vi "Read Com.vi"() -> ()   [LabVIEW 2016]
panel:
  in  "Boolean":bool
  out "Waveform Chart":dbl(graph)
  in  "stop":bool
  out "concatenated string":string
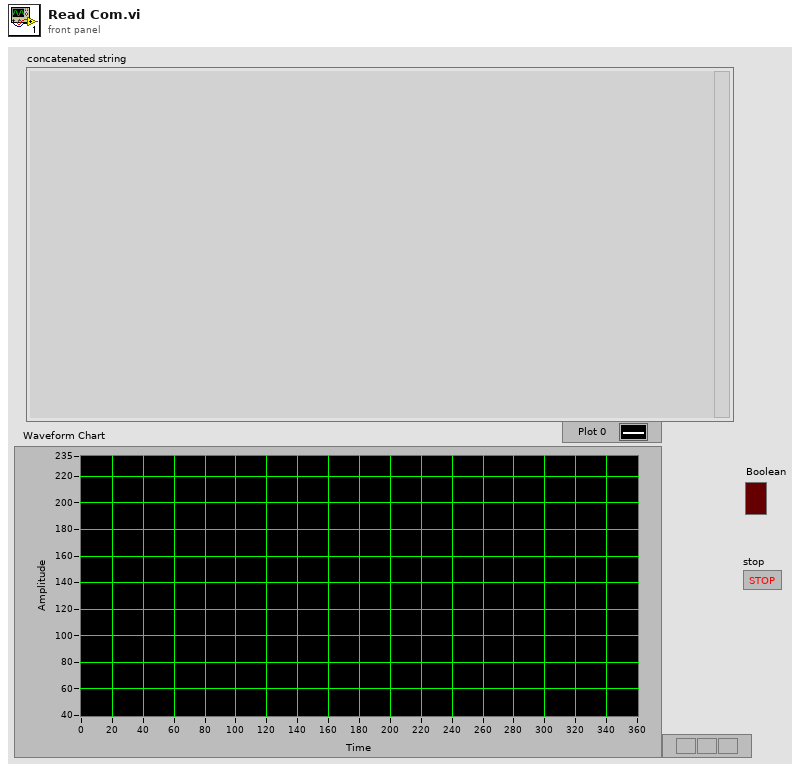
[diagram p1: front panel]
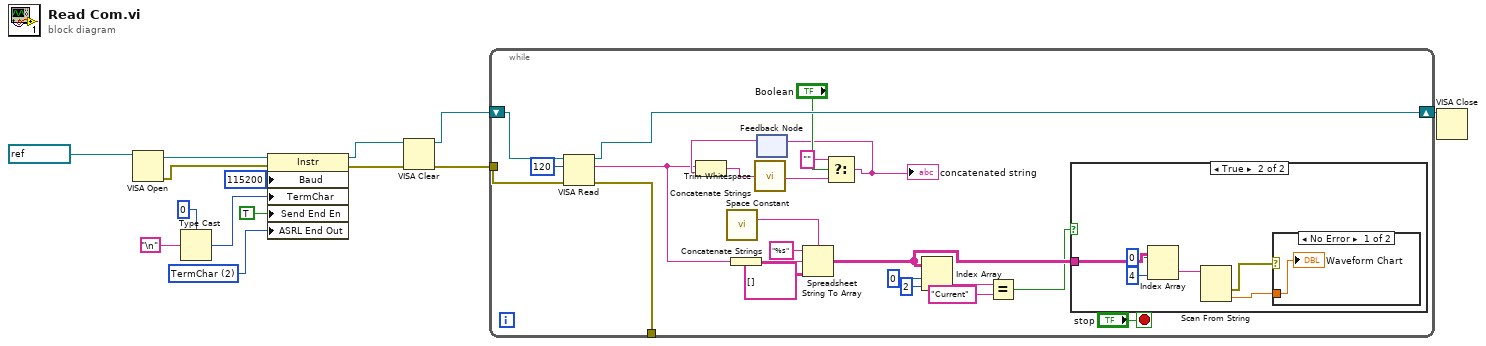
[diagram p0: block diagram]
diagram:
  w4 = u16 2 items=["None", "Last Bit", "TermChar", "Break"] ("Serial Settings:End Mode for Writes")
  n1 = VISA Open(VISA resource name=refnum<visa-resource-name> "COM3") -> (VISA resource name=w13:refnum<visa-resource-name>, error out=w10:errorcluster)  [unwired: 4 in]
  n2 = Type Cast(type=u8 0 ("Message Based Settings:Termination Character"), x="\n") -> (*(type *) &x=w7:u8)
  n3 = property class="Instr"(reference=w13, error in=w10, "Baud"=u32 115200 ("Serial Settings:Baud Rate"), "TermChar"=w7, "Send End En"=TRUE ("Message Based Settings:Send End Enable"), "ASRL End Out"=w4) -> (reference out=w2:refnum<visa-resource-name>, error out=w11:errorcluster)
  n4 = VISA Clear(VISA resource name=w2, error in (no error)=w11) -> (VISA resource name out=w1:refnum<visa-resource-name>, error out=w3:errorcluster)
  n5 = while {
    tunnel: w3 -> [w35]
    shift-right: [w34] -> w9
    shift-left: w1 -> [w37]
    tunnel: [w21] -> _
    stop <- "stop" stop-if-true
    n6 = VISA Read(VISA resource name=w37, byte count=u32 120, error in (no error)=w35) -> (VISA resource name out=w34:refnum<visa-resource-name>, read buffer=w31:string, error out=w21:errorcluster)  [unwired: 1 out]
    n7 = call <vilib>:"Space Constant.vi"() -> ("String"=w27:string)
    n8 = Concatenate Strings(w31) -> (w30:string)
    n9 = feedback #1() -> (w32:string)  [unwired: 1 in]
    n10 = Concatenate Strings(w31, w32) -> (w36:string)
    n11 = call <vilib>:"Trim Whitespace.vi"("string"=w36) -> ("trimmed string"=w25:string)  [unwired: 1 in]
    n12 = Spreadsheet String To Array(delimiter (Tab)=w27, format string="%s", spreadsheet string=w30, array type (2D Dbl)=string[][] []) -> (array=w20:string[][])
    n13 = Select(t="", s="Boolean", f=w25) -> (s? t:f=w23:string)
    "concatenated string" <- w23
    n14 = feedback-in #1(w23) -> ()
    n15 = Index Array(array=w20, index (row)=0 ("disabled index (row)"), index (col)=2 ("disabled index (col)")) -> (element=w17:string)
    n16 = Equal?(x=w17, y="Current") -> (x = y?=w15:bool)
    n17 = case shown="True" w15 {
      tunnel: w20 -> [_ w43]
      frame False {
      }
      frame True {
        n18 = Index Array(array=w43, index (row)=0 ("disabled index (row)"), index (col)=4 ("disabled index (col)")) -> (element=w40:string)
        n19 = Scan From String(input string=w40) -> (error out=w39:errorcluster, output 1=w38:dbl)  [unwired: 4 in, 2 out]
        n20 = case shown="No Error" w39 {
          tunnel: w38 -> [w44 _]
          frame No Error {
            "Waveform Chart" <- w44
          }
          frame Error {
          }
        }
      }
    }
  }
  n21 = VISA Close(VISA resource name=w9) -> ()  [unwired: 1 in, 1 out]
